vi "Live Capture Functional Stack3.64bit.Test.vi"() -> ()   [LabVIEW 2014]
uses:
  subvis/Stack Track.ctl
  subvis/Stack_State.ctl
  Desktop/camtiff/ctiff.llb/__CTIFFNewFileAndStyleUINT16.vi
  Desktop/camtiff/ctiff.llb/__CTIFFAddNewPageUINT16.vi
panel:
  out "Frame Index":i32
  in  "Temp":path=path "C:/temp.tmp"
  in  "Frames":i32=100
  in  "HardDisk Record":bool
  in  "Internal Line Interval":dbl
  in  "Slit Width / Lines":sgl=150.0
  in  "Camera Readout Mode":u16(ring)=12 items=["Full Frame"=1, "Slit Scanning"=12]
  in  "Readout Direction":sgl(ring)=1.0 items=["Forward"=1, "Backward"=2]
  in  "Trigger Mode":sgl(ring)=1.0 items=["Normal"=1, "Start "=6]
  in  "Trigger Source":sgl(ring)=2.0 items=["Internal"=1, "External"=2]
  out "State":T1=enum."Start Sequence"
  out "Image":u16[][](graph)
  out "Saving":bool
  in  "AutoIncrement":bool=TRUE
  in  "Path":path=path "C:/Users/spim/Desktop/Craig Cap/temp/a.tiff"
  in  "Frames":i32=100
  out "Frame Index":i32
  out "error out":errorcluster
  in  "stop":bool
  in  "Ram Record":bool
  out "Total Frames":i32
  out "Elapsed Time":u32
  out "Software FPS":dbl
  out "Camera FPS":dbl
  in  "H Offset":i32 min=0 max=0 step=4
  in  "H Width":i32 min=0 max=2048 step=4
  out "SMD":dbl
  out "SHO":i32
  in  "V Offset":i32 min=0 max=0 step=4
  in  "V Width":i32 min=0 max=2048 step=4
  in  "Binning":u16(ring) items=["1x1"=1, "2x2"=2, "4x4"=4]
  out "SHW":i32
  out "SVO":i32
  out "SVW":i32
  in  "Scan Mode":dbl min=0.0 max=2.0 step=1.0
  in  "Exposure":dbl min=0.0 max=10.000004210526315 step=1e-08
  out "EXP":dbl
  out "Camera Model":string
  out "Camera Version":string
  out "Camera Serial":string
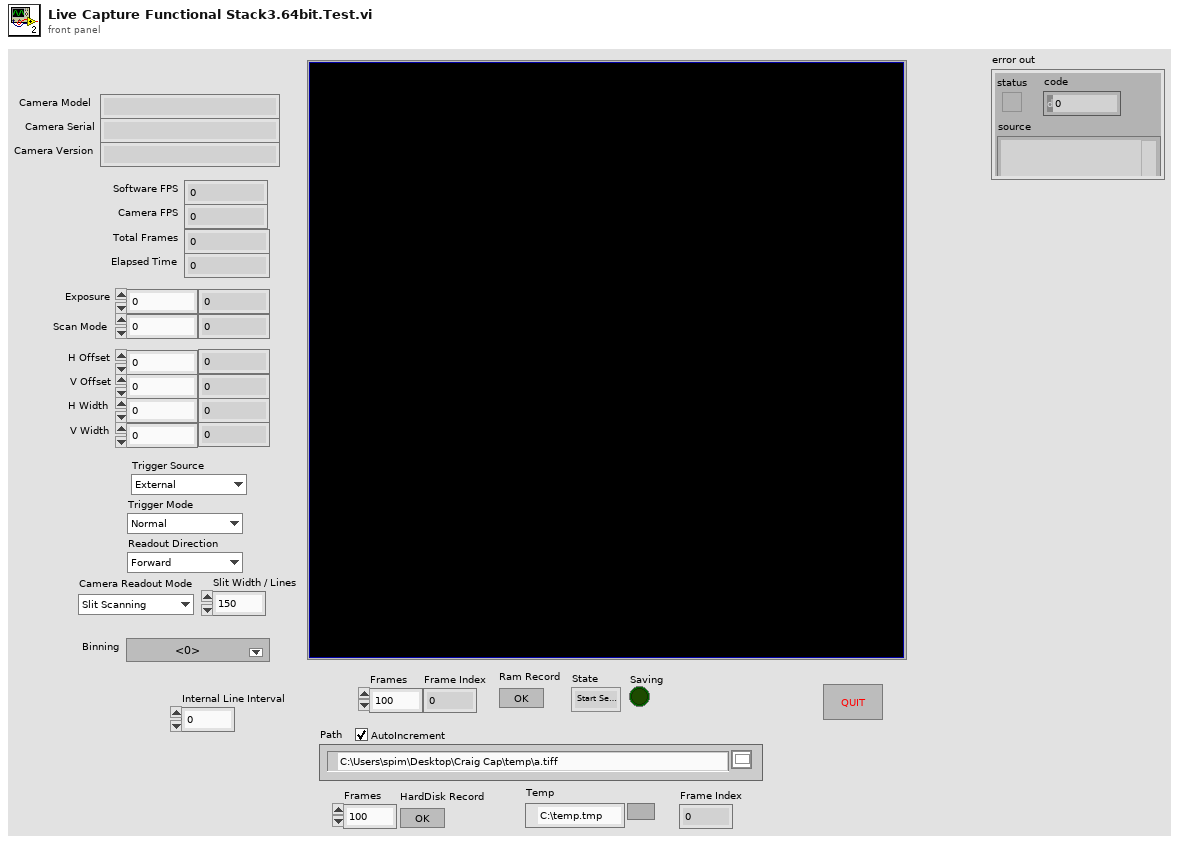
[diagram p1: front panel]
types:
  T1 = typedef "Stack Track.ctl" = enum16{"Idle", "Start Sequence", "Read Disk", "STOP", "Collecting", "End"}
  T2 = enum8{"Enabled", "Disabled", "Disabled and Grayed Out"}
  T3 = typedef "Stack_State.ctl" = cluster{"State":T1, "Stack Number":i32, "Image":u16[][]}
  T4 = cluster{"Model":string, "Camera ID":string, "Firmware":string}
  T5 = cluster{"Value":i32, "Minimum":i32, "Maximum":i32, "Increment":i32}
  T6 = cluster{"height":u32, "width":u32, "datatype":u32}
  T7 = cluster{"H Offset":i32, "V Offset":i32, "H Width":i32, "V Width":i32}
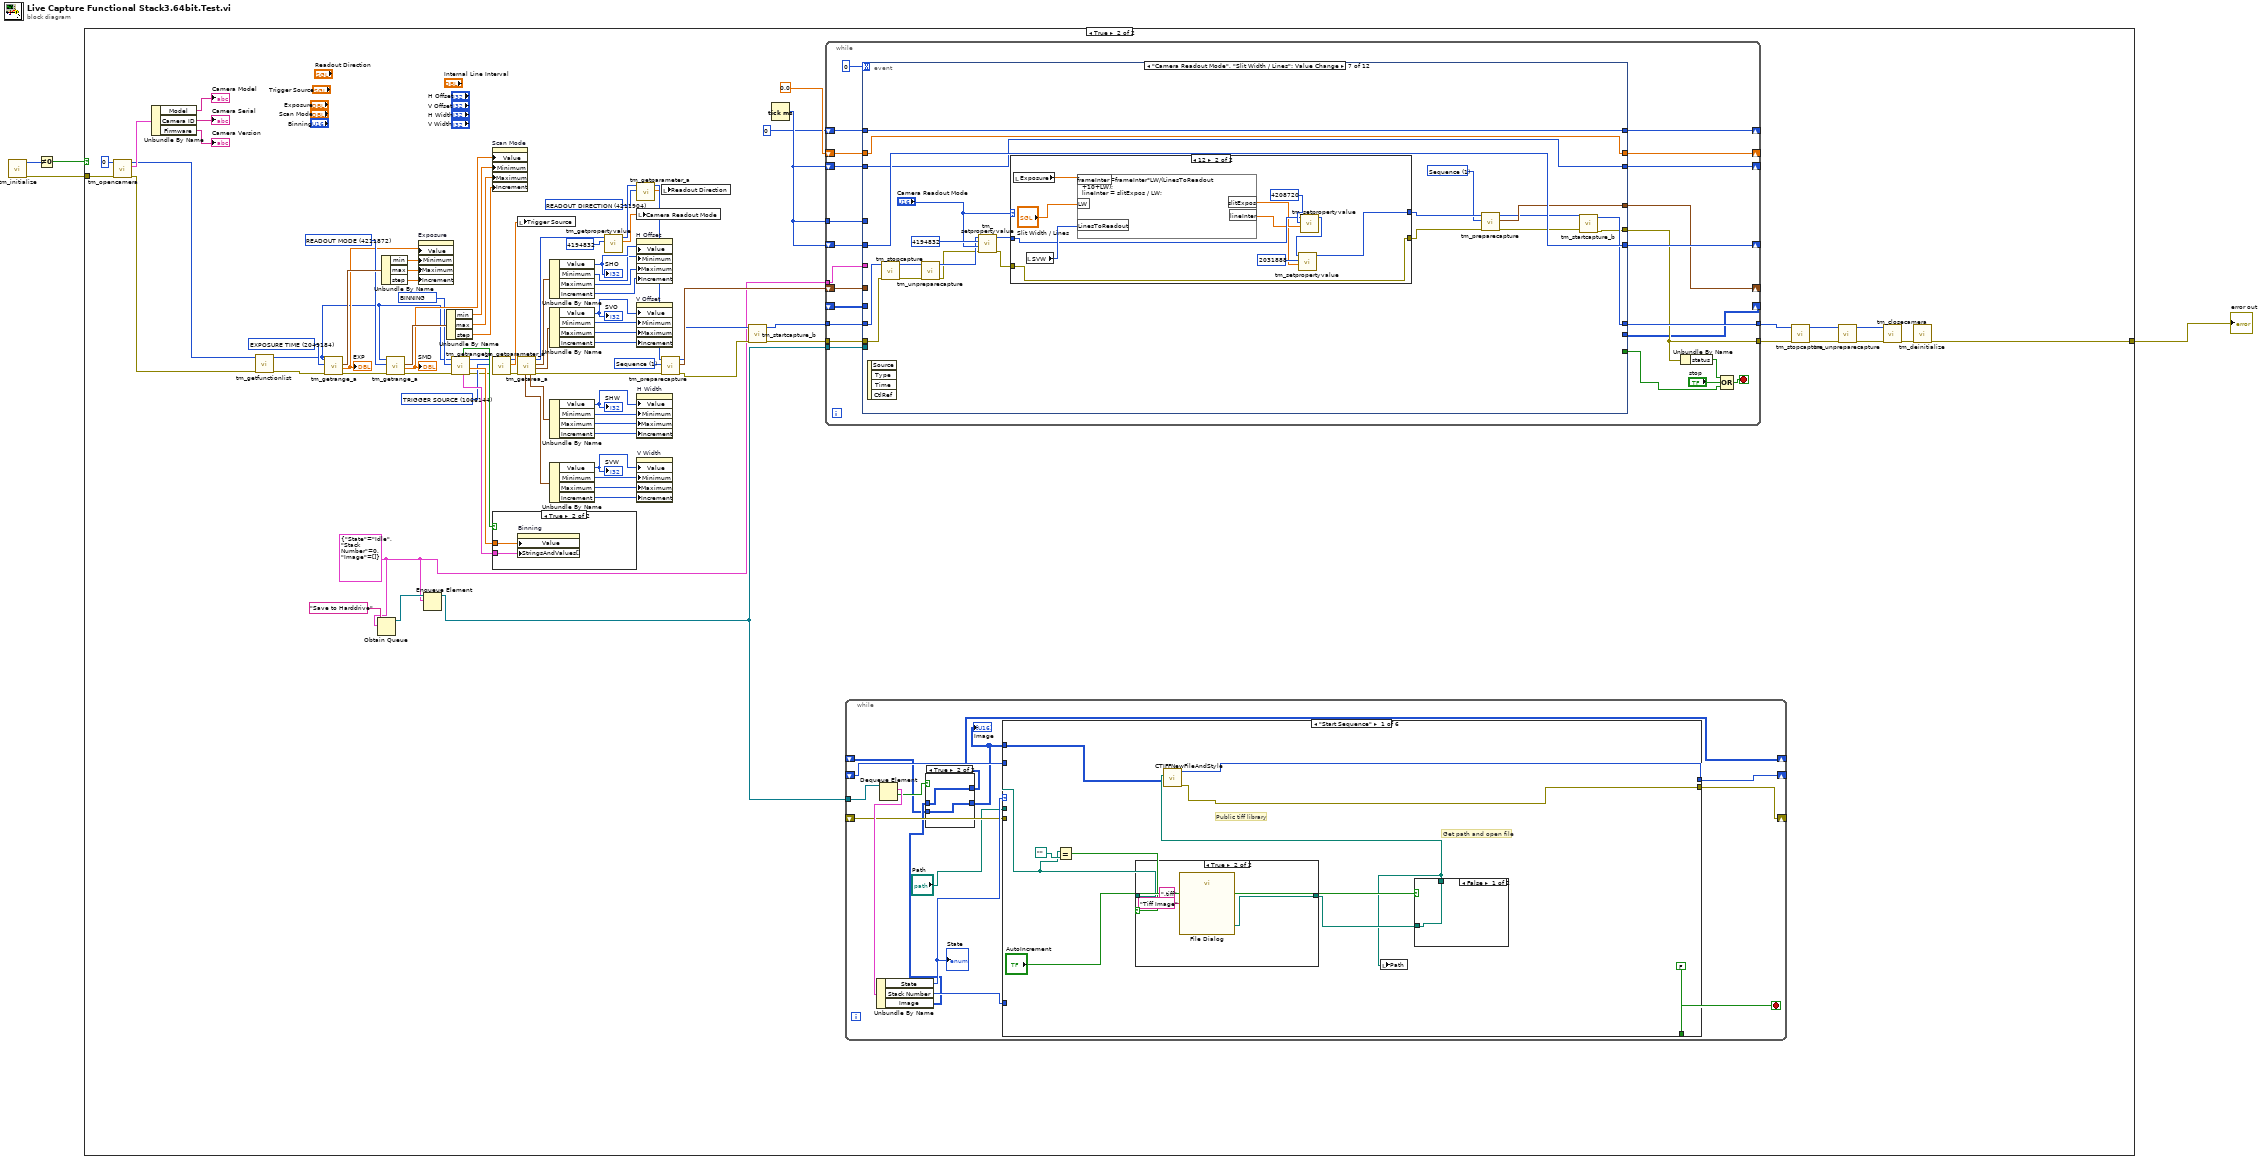
[diagram p0: block diagram]
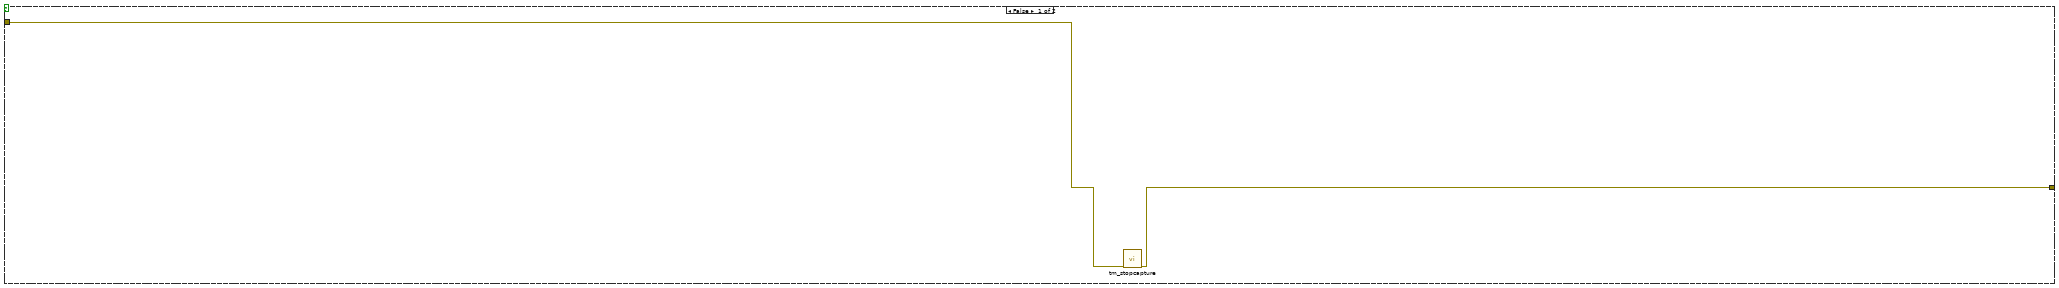
[diagram p2: hidden frame]
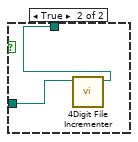
[diagram p5: hidden frame]
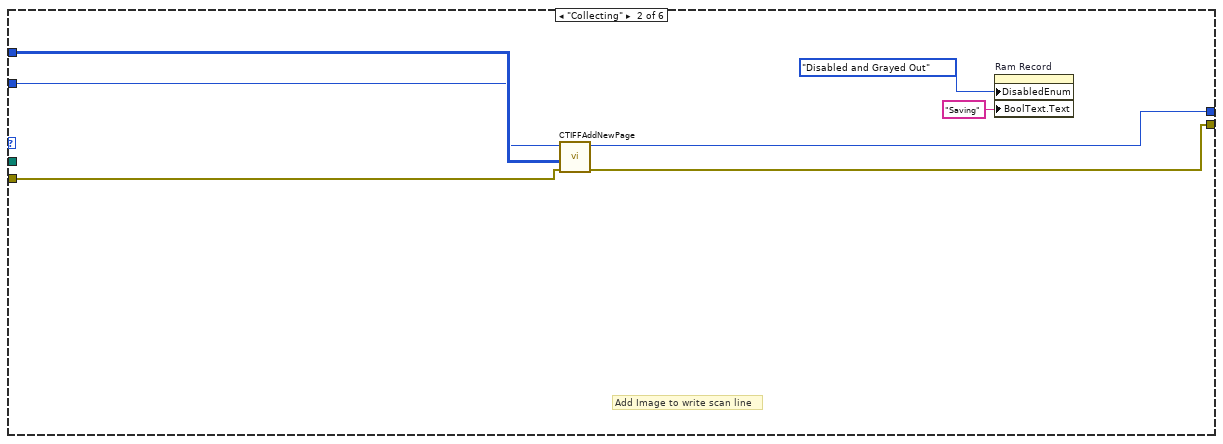
[diagram p6: hidden frame]
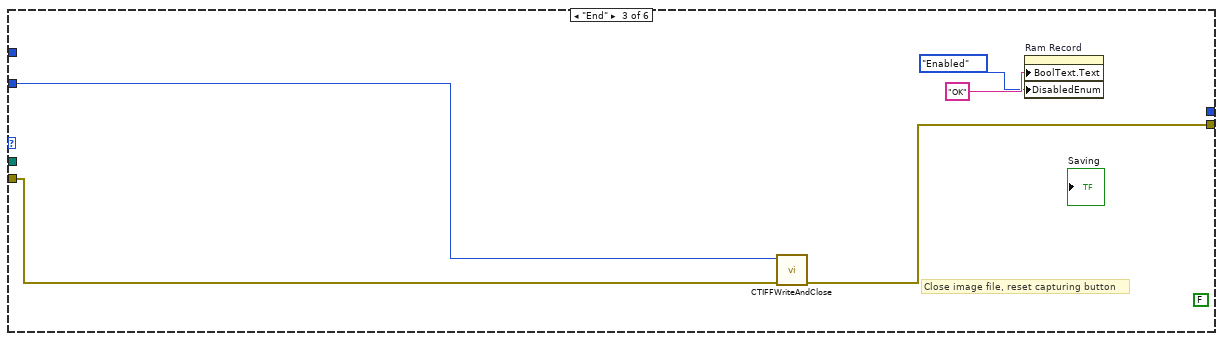
[diagram p7: hidden frame]
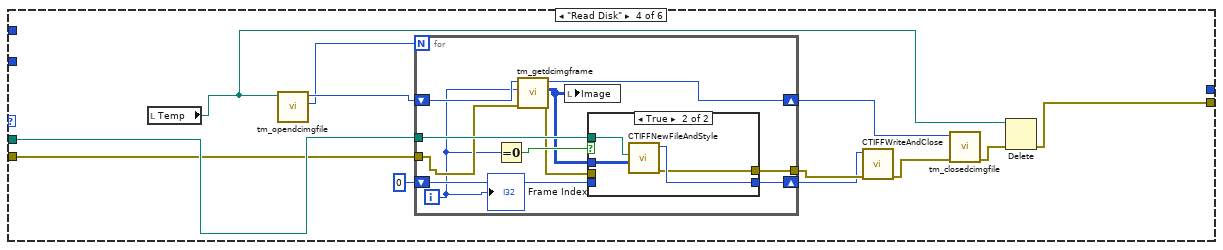
[diagram p8: hidden frame]
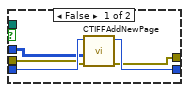
[diagram p9: hidden frame]
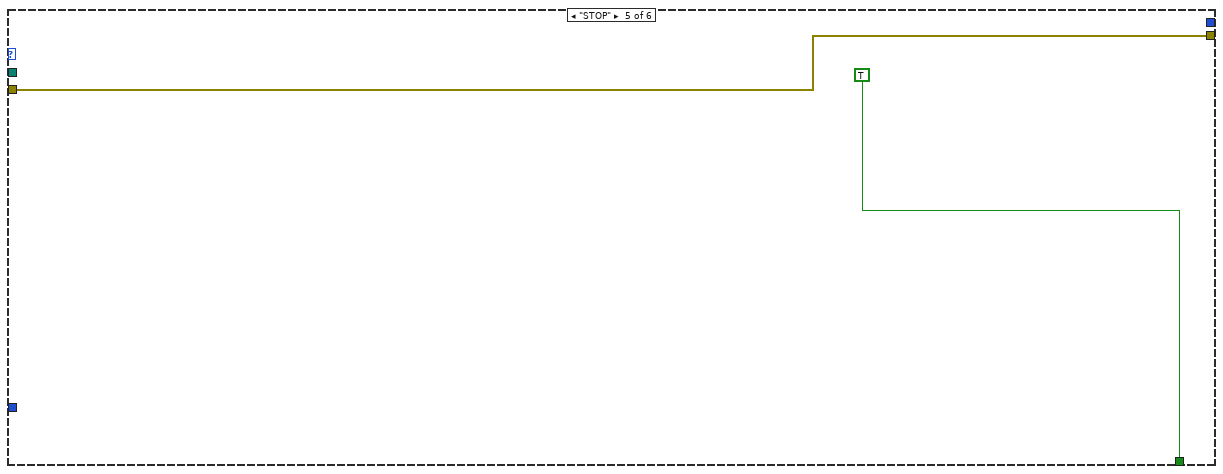
[diagram p10: hidden frame]
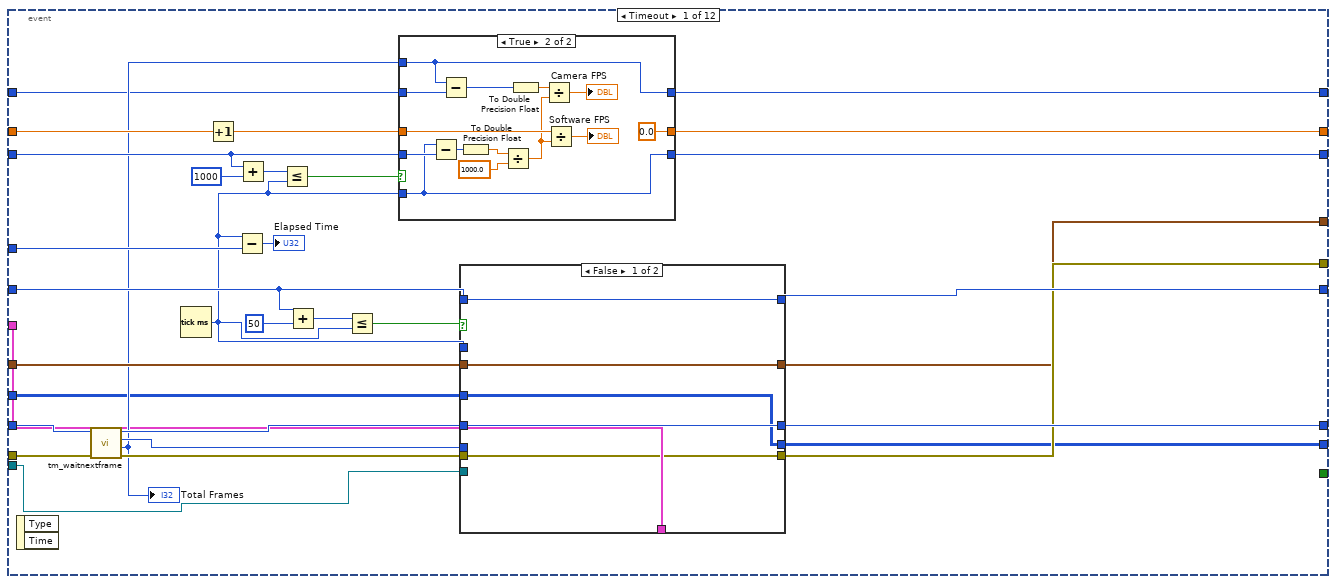
[diagram p13: hidden frame]
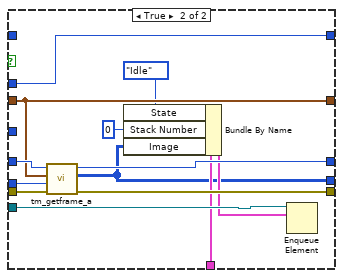
[diagram p15: hidden frame]
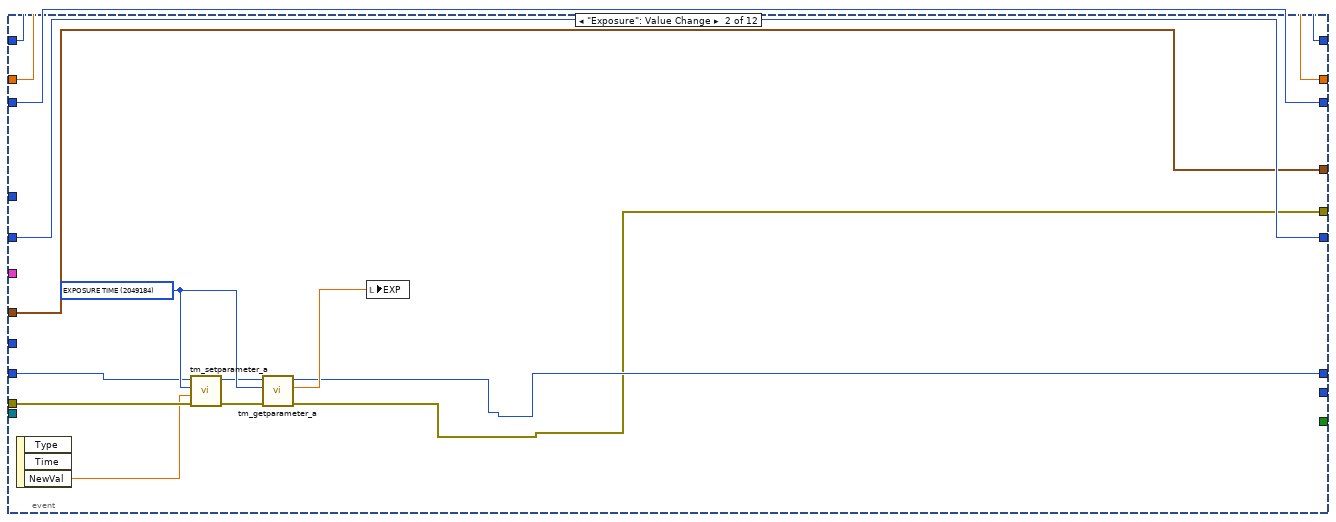
[diagram p16: hidden frame]
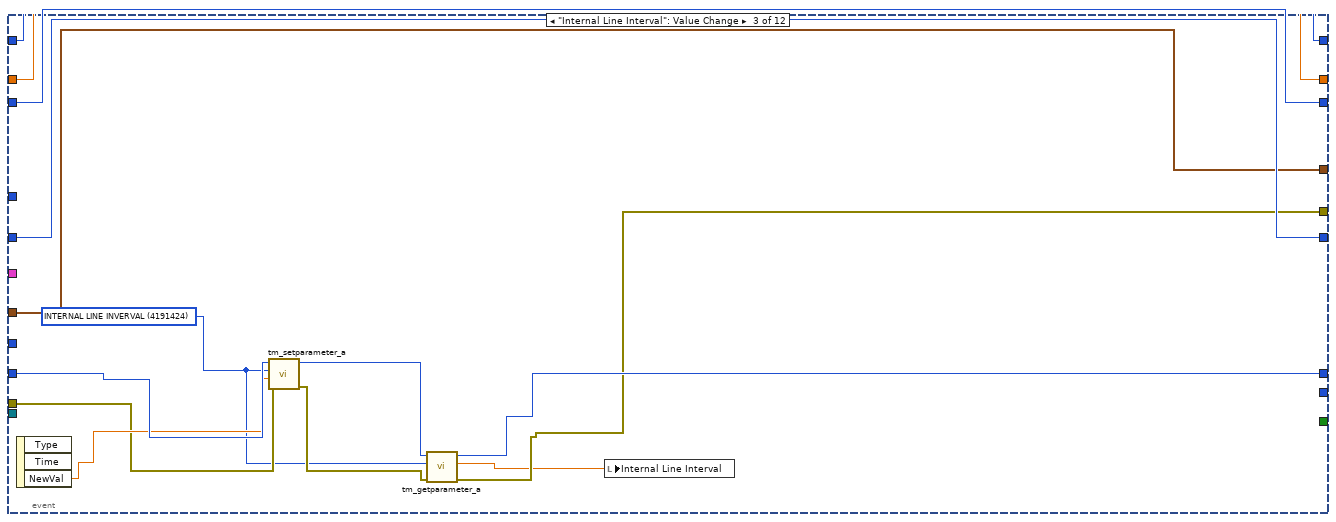
[diagram p17: hidden frame]
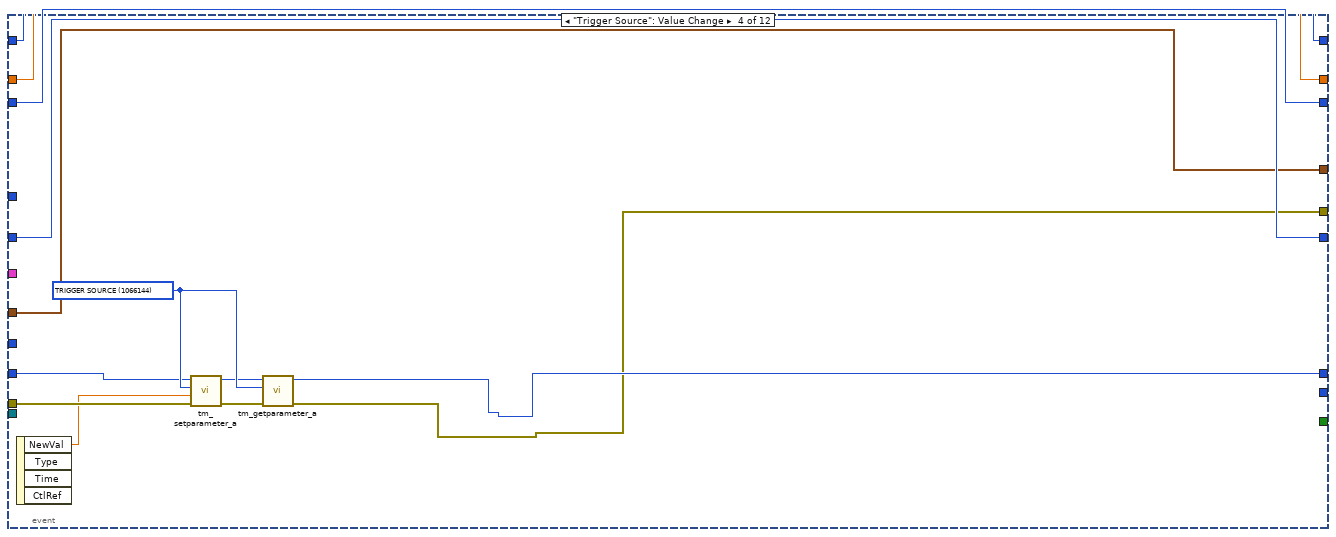
[diagram p18: hidden frame]
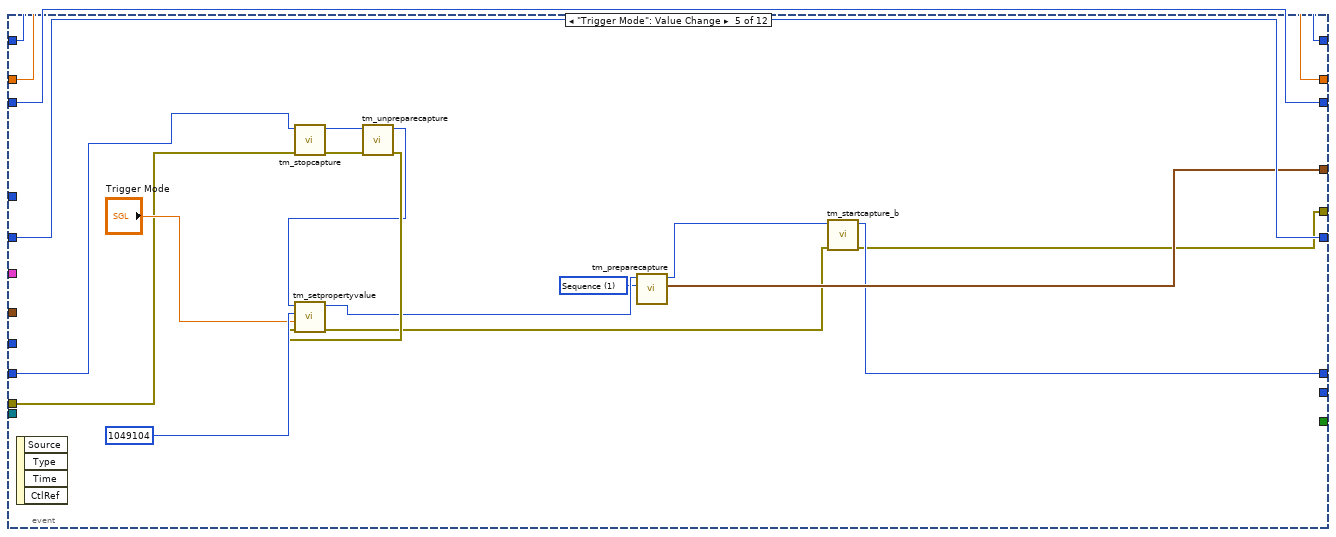
[diagram p19: hidden frame]
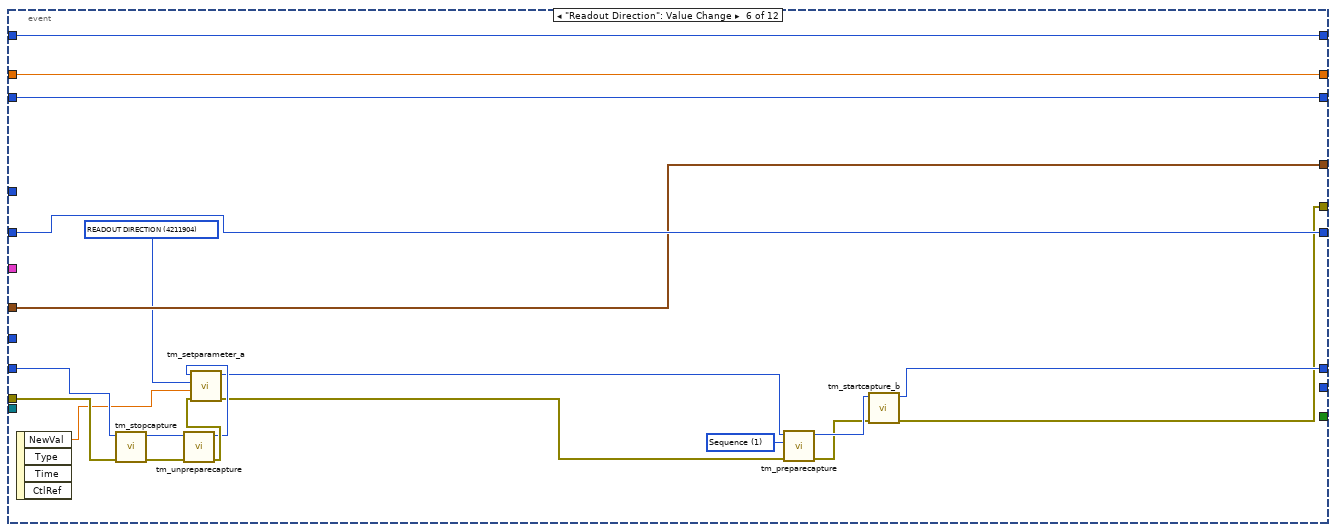
[diagram p20: hidden frame]
diagram:
  n1 = call <userlib>:"tm_initialize.vi"() -> ("error out"=w2:errorcluster, "Number Of Cameras"=w1:u32)  [unwired: 8 in, 2 out]
  n2 = Not Equal To 0?(x=w1) -> (x != 0?=w4:bool)
  n3 = case shown="True" w4 {
    tunnel: [w5 w86] -> w3
    tunnel: w2 -> [w6 w89]
    frame False {
      n4 = call <userlib>:"tm_stopcapture.vi"("error in (no error)"=w6) -> ("error out"=w5:errorcluster)  [unwired: 9 in, 1 out]
    }
    frame True {
      w14 = u32 4211904 items=["SENSOR MODE"=4212128, "CCD MODE"=4212384, "READOUT MODE"=4211872, "ACTIVE VIEW INDEX"=4343136, "BITS PER CHANNEL"=4342976, "IMAGE PIXEL TYPE"=4343296, "BINNING"=4215968, "EXPOSURE TIME"=2049184, "CONTRAST GAIN"=3163312, "CONTRAST OFFSET"=3163328, "LIGHT MODE"=2114720, "SENSITIVITY"=2114992, "PHOTON IMAGING MODE"=2115200, "HIGH DYNAMIC RANGE MODE"=3163360, "WHITE BALANCE"=3163568, "TEMPERATURE"=2115232, "TEMPERATURE TARGET"=2115264, "SENSOR COOLER FAN"=2115296, "LINEBUNDLE HEIGHT"=4212192, "MECHANICAL SHUTTER"=2115488, "BACK FOCUS POSITION"=8422304, "TRIGGER CONNECTOR"=1066432, "TRIGGER SOURCE"=1066144, "OUTPUT TRIGGER SOURCE"=1852576, "TRIGGER GLOBAL EXPOSURE"=2049680, "FIRST TRIGGER BEHAVIOR"=2049696, "CHANNEL SYNC"=1852352, "READOUT DIRECTION"=4211904, "PRE HSYNC COUNT"=1852704] ("Parameter")
      w24 = u32 1066144 items=["SENSOR MODE"=4212128, "CCD MODE"=4212384, "READOUT MODE"=4211872, "ACTIVE VIEW INDEX"=4343136, "BITS PER CHANNEL"=4342976, "IMAGE PIXEL TYPE"=4343296, "BINNING"=4215968, "EXPOSURE TIME"=2049184, "CONTRAST GAIN"=3163312, "CONTRAST OFFSET"=3163328, "LIGHT MODE"=2114720, "SENSITIVITY"=2114992, "PHOTON IMAGING MODE"=2115200, "HIGH DYNAMIC RANGE MODE"=3163360, "WHITE BALANCE"=3163568, "TEMPERATURE"=2115232, "TEMPERATURE TARGET"=2115264, "SENSOR COOLER FAN"=2115296, "LINEBUNDLE HEIGHT"=4212192, "MECHANICAL SHUTTER"=2115488, "BACK FOCUS POSITION"=8422304, "TRIGGER CONNECTOR"=1066432, "TRIGGER SOURCE"=1066144, "OUTPUT TRIGGER SOURCE"=1852576, "TRIGGER GLOBAL EXPOSURE"=2049680, "FIRST TRIGGER BEHAVIOR"=2049696, "CHANNEL SYNC"=1852352, "READOUT DIRECTION"=4211904, "PRE HSYNC COUNT"=1852704] ("Parameter")
      w7 = T3 {"State"=enum."Idle", "Stack Number"=0, "Image"=[]} ("input cluster")
      w32 = u32 2049184 items=["BINNING"=4215968, "BITS PER CHANNEL"=4342976, "ACTIVE VIEW INDEX"=4343136, "CCD MODE"=4212384, "SENSOR MODE"=4212128, "READOUT MODE"=4211872, "EXPOSURE TIME"=2049184, "CONTRAST GAIN"=3163312, "CONTRAST OFFSET"=3163328, "LIGHT MODE"=2114720, "SENSITIVITY"=2114992, "WHITE BALANCE"=3163568, "PHOTON IMAGING MODE"=2115200, "HIGH DYNAMIC RANGE MODE"=3163360, "TRIGGER SOURCE"=1066144, "TRIGGER ACTIVE"=1066160, "TRIGGER MODE"=1066400, "TRIGGER POLARITY"=1066416, "TRIGGER GLOBAL EXPOSURE"=2049680, "FIRST TRIGGER BEHAVIOR"=2049696, "TRIGGER TIMES"=1066448, "OUTPUT TRIGGER POLARITY"=1852592, "OUTPUT TRIGGER DELAY"=1852624, "OUTPUT TRIGGER PERIOD"=1852640, "TEMPERATURE"=2115232, "TEMPERATURE TARGET"=2115264, "SENSOR COOLER FAN"=2115296, "MECHANICAL SHUTTER"=2115488, "BACK FOCUS POSITION"=8422304, "FRAMEBUNDLE MODE"=4346784, "FRAMEBUNDLE NUMBER"=4346800, "LINEBUNDLE HEIGHT"=4212192, "TRIGGER CONNECTOR"=1066432, "IMAGE PIXEL TYPE"=4343296, "OUTPUT TRIGGER KIND"=1852656, "READOUT DIRECTION"=4211904, "CHANNEL SYNC"=1852352] ("Parameter")
      w33 = u32 4211872 items=["BINNING"=4215968, "BITS PER CHANNEL"=4342976, "ACTIVE VIEW INDEX"=4343136, "CCD MODE"=4212384, "SENSOR MODE"=4212128, "READOUT MODE"=4211872, "EXPOSURE TIME"=2049184, "CONTRAST GAIN"=3163312, "CONTRAST OFFSET"=3163328, "LIGHT MODE"=2114720, "SENSITIVITY"=2114992, "WHITE BALANCE"=3163568, "PHOTON IMAGING MODE"=2115200, "HIGH DYNAMIC RANGE MODE"=3163360, "TRIGGER SOURCE"=1066144, "TRIGGER ACTIVE"=1066160, "TRIGGER MODE"=1066400, "TRIGGER POLARITY"=1066416, "TRIGGER GLOBAL EXPOSURE"=2049680, "FIRST TRIGGER BEHAVIOR"=2049696, "TRIGGER TIMES"=1066448, "OUTPUT TRIGGER POLARITY"=1852592, "OUTPUT TRIGGER DELAY"=1852624, "OUTPUT TRIGGER PERIOD"=1852640, "TEMPERATURE"=2115232, "TEMPERATURE TARGET"=2115264, "SENSOR COOLER FAN"=2115296, "MECHANICAL SHUTTER"=2115488, "BACK FOCUS POSITION"=8422304, "FRAMEBUNDLE MODE"=4346784, "FRAMEBUNDLE NUMBER"=4346800, "LINEBUNDLE HEIGHT"=4212192, "TRIGGER CONNECTOR"=1066432, "IMAGE PIXEL TYPE"=4343296, "OUTPUT TRIGGER KIND"=1852656, "READOUT DIRECTION"=4211904, "CHANNEL SYNC"=1852352] ("Parameter")
      w34 = u32 4215968 items=["BINNING"=4215968, "BITS PER CHANNEL"=4342976, "ACTIVE VIEW INDEX"=4343136, "CCD MODE"=4212384, "SENSOR MODE"=4212128, "READOUT MODE"=4211872, "EXPOSURE TIME"=2049184, "CONTRAST GAIN"=3163312, "CONTRAST OFFSET"=3163328, "LIGHT MODE"=2114720, "SENSITIVITY"=2114992, "WHITE BALANCE"=3163568, "PHOTON IMAGING MODE"=2115200, "HIGH DYNAMIC RANGE MODE"=3163360, "TRIGGER SOURCE"=1066144, "TRIGGER ACTIVE"=1066160, "TRIGGER MODE"=1066400, "TRIGGER POLARITY"=1066416, "TRIGGER GLOBAL EXPOSURE"=2049680, "FIRST TRIGGER BEHAVIOR"=2049696, "TRIGGER TIMES"=1066448, "OUTPUT TRIGGER POLARITY"=1852592, "OUTPUT TRIGGER DELAY"=1852624, "OUTPUT TRIGGER PERIOD"=1852640, "TEMPERATURE"=2115232, "TEMPERATURE TARGET"=2115264, "SENSOR COOLER FAN"=2115296, "MECHANICAL SHUTTER"=2115488, "BACK FOCUS POSITION"=8422304, "FRAMEBUNDLE MODE"=4346784, "FRAMEBUNDLE NUMBER"=4346800, "LINEBUNDLE HEIGHT"=4212192, "TRIGGER CONNECTOR"=1066432, "IMAGE PIXEL TYPE"=4343296, "OUTPUT TRIGGER KIND"=1852656, "READOUT DIRECTION"=4211904, "CHANNEL SYNC"=1852352] ("Parameter")
      w84 = 1 items=["Snap", "Sequence"] ("Capture mode")
      n5 = call <userlib>:"tm_opencamera.vi"("error in (no error)"=w89, "Camera Index"=u32 0) -> ("error out"=w28:errorcluster, "Camera Details"=w46:T4, "Handle out"=w12:u32)  [unwired: 7 in]
      n6 = Unbundle By Name(w46) -> ("Model"=→"Camera Model":string, "Camera ID"=→"Camera Serial":string, "Firmware"=→"Camera Version":string)
      n7 = call <userlib>:"tm_getfunctionlist.vi"("error in (no error)"=w28, "Handle in"=w12) -> ("error out"=w27:errorcluster, "Handle out"=w29:u32)  [unwired: 7 in, 1 out]
      n8 = call <userlib>:"tm_getrange_a.vi"("error in (no error)"=w27, "Parameter"=w32, "Handle in"=w29) -> ("error out"=w41:errorcluster, "default"=w30:dbl, "Range"=w42:cluster{"min":dbl, "max":dbl, "step":dbl})  [unwired: 2 in, 4 out]
      "EXP" <- w30
      n9 = Obtain Queue(name (unnamed)="Save to Harddrive", element data type=w7) -> (queue out=w9:refnum<queue>)  [unwired: 3 in, 2 out]
      n10 = Unbundle By Name(w42) -> ("min"=w79:dbl, "max"=w78:dbl, "step"=w77:dbl)
      n11 = call <userlib>:"tm_getrange_a.vi"("error in (no error)"=w41, "Parameter"=w33, "Handle in"=w29) -> ("error out"=w38:errorcluster, "default"=w39:dbl, "Range"=w40:cluster{"min":dbl, "max":dbl, "step":dbl})  [unwired: 2 in, 4 out]
      "SMD" <- w39
      n12 = property on="Exposure" class="DigNum (strict)"("Value"=w30, "Minimum"=w79, "Maximum"=w78, "Increment"=w77) -> ()  [unwired: 2 in, 2 out]
      n13 = Enqueue Element(queue=w9, element=w7) -> (queue out=w8:refnum<queue>)  [unwired: 2 in, 2 out]
      n14 = Unbundle By Name(w40) -> ("min"=w76:dbl, "max"=w75:dbl, "step"=w74:dbl)
      n15 = call <userlib>:"tm_getrange_a.vi"("error in (no error)"=w38, "Parameter"=w34, "Handle in"=w29) -> ("error out"=w21:errorcluster, "default"=w36:dbl, "Handle out"=w23:u32, "Value Names"=w35:cluster{"Name":string, "Value":dbl}[], "Writable"=w37:bool)  [unwired: 2 in, 2 out]
      n16 = property on="Scan Mode" class="DigNum (strict)"("Value"=w39, "Minimum"=w76, "Maximum"=w75, "Increment"=w74) -> ()  [unwired: 2 in, 2 out]
      n17 = call <userlib>:"tm_getparameter_a.vi"("error in (no error)"=w21, "Parameter"=w24, "Handle in"=w23) -> ("error out"=w20:errorcluster, "Value out"=w25:dbl, "Handle out"=w22:u32)  [unwired: 6 in]
      n18 = case shown="True" w37 {
        tunnel: w35 -> [_ w174]
        tunnel: w36 -> [_ w173]
        frame False {
        }
        frame True {
          n19 = property on="Binning" class="Ring (strict)"("Value"=w173, "StringsAndValues[]"=w174) -> ()  [unwired: 2 in, 2 out]
        }
      }
      n20 = local write "Trigger Source"(w25) -> ()
      n21 = call <userlib>:"tm_getarea_a.vi"("error in (no error)"=w20, "Handle in"=w22) -> ("error out"=w26:errorcluster, "V Offset"=w73:T5, "H Offset"=w52:T5, "Handle out"=w17:u32, "H Width"=w72:T5, "V Width"=w71:T5)  [unwired: 4 in]
      n22 = Unbundle By Name(w52) -> ("Value"=w51:i32, "Minimum"=w50:i32, "Maximum"=w49:i32, "Increment"=w48:i32)
      "SHO" <- w51
      n23 = Unbundle By Name(w73) -> ("Value"=w61:i32, "Minimum"=w70:i32, "Maximum"=w69:i32, "Increment"=w68:i32)
      "SVO" <- w61
      n24 = Unbundle By Name(w72) -> ("Value"=w60:i32, "Minimum"=w67:i32, "Maximum"=w66:i32, "Increment"=w65:i32)
      "SHW" <- w60
      n25 = Unbundle By Name(w71) -> ("Value"=w59:i32, "Minimum"=w64:i32, "Maximum"=w63:i32, "Increment"=w62:i32)
      "SVW" <- w59
      n26 = call <userlib>:"tm_getpropertyvalue.vi"("Property ID"=u32 4194832, "Handle in"=w17) -> ("Value in"=w18:sgl, "Handle out"=w16:u32)  [unwired: 7 in, 1 out]
      n27 = call <userlib>:"tm_getparameter_a.vi"("Parameter"=w14, "Handle in"=w16) -> ("Value out"=w13:dbl, "Handle out"=w15:u32)  [unwired: 7 in, 1 out]
      n28 = local write "Camera Readout Mode"(w18) -> ()
      n29 = property on="H Offset" class="DigNum (strict)"("Value"=w51, "Minimum"=w50, "Maximum"=w49, "Increment"=w48) -> ()  [unwired: 2 in, 2 out]
      n30 = property on="V Offset" class="DigNum (strict)"("Value"=w61, "Minimum"=w70, "Maximum"=w69, "Increment"=w68) -> ()  [unwired: 2 in, 2 out]
      n31 = property on="H Width" class="DigNum (strict)"("Value"=w60, "Minimum"=w67, "Maximum"=w66, "Increment"=w65) -> ()  [unwired: 2 in, 2 out]
      n32 = property on="V Width" class="DigNum (strict)"("Value"=w59, "Minimum"=w64, "Maximum"=w63, "Increment"=w62) -> ()  [unwired: 2 in, 2 out]
      n33 = local write "Readout Direction"(w13) -> ()
      n34 = call <userlib>:"tm_preparecapture.vi"("error in (no error)"=w26, "Capture mode"=w84, "Handle in"=w15) -> ("error out"=w10:errorcluster, "Buffer Info"=w81:T6, "Handle out"=w11:u32)  [unwired: 5 in, 1 out]
      n35 = call <userlib>:"tm_startcapture_b.vi"("error in (no error)"=w10, "Handle in"=w11) -> ("error out"=w83:errorcluster, "Handle out"=w82:u32)  [unwired: 8 in]
      n36 = Tick Count (ms)() -> (millisecond timer value=w80:u32)
      n37 = while {
        tunnel: w83 -> [w187]
        tunnel: [w185] -> w58
        tunnel: [w184] -> w57
        shift-right: [w194] -> _
        shift-left: w80 -> [w192]
        shift-right: [w195] -> _
        shift-left: 0.0 -> [w193]
        shift-right: [w186] -> _
        shift-left: w80 -> [w190]
        tunnel: w82 -> [w188]
        tunnel: w80 -> [w191]
        shift-right: [w183] -> _
        shift-left: w81 -> [w189]
        shift-right: [w180] -> _
        shift-left: 0 -> [w181]
        tunnel: w8 -> [w179]
        shift-right: [w177] -> _
        shift-left: _ -> [w176]
        tunnel: w7 -> [w175]
        stop <- w196 stop-if-true
        n38 = event shown="[6] \"Camera Readout Mode\", \"Slit Width / Lines\": Value Change" {
          selector: _ -> [_ _ _ _ _ _ _ _ _ _ _ _]
          dyn-events: _ -> [_ _ _ _ _ _ _ _ _ _ _ _]
          timeout: 0 -> [_ _ _ _ _ _ _ _ _ _ _ _]
          tunnel: [w208 w277 w291 w304 w323 w343 w365 w393 w490 w584 w620 w665] -> w195
          tunnel: [w207 w278 w292 w305 w324 w344 w366 w394 w491 w585 w621 w666] -> w194
          tunnel: w193 -> [w219 w277 w291 w304 w323 w343 w365 w393 w490 w584 w620 w665]
          tunnel: w192 -> [w210 w278 w292 w305 w324 w344 w366 w394 w491 w585 w621 w666]
          tunnel: w191 -> [w215 _ _ _ _ _ _ _ _ _ _ _]
          tunnel: w190 -> [w220 w279 w293 w306 w325 w345 w367 w389 w486 w586 w628 w673]
          tunnel: w189 -> [w214 w276 w290 w303 _ w342 _ w390 w487 _ _ _]
          tunnel: w188 -> [w222 w271 w285 w299 w317 w336 w358 w397 w494 w581 w597 w635]
          tunnel: w187 -> [w221 w273 w281 w300 w316 w339 w357 w398 w495 w580 w596 w634]
          tunnel: [w218 w279 w293 w306 w325 w345 w367 w389 w486 w586 w628 w673] -> w186
          tunnel: [w217 w267 w288 w296 w308 w329 w348 w395 w492 w575 w623 w668] -> w185
          tunnel: [w216 w266 w287 w295 w307 w328 w346 w396 w493 w576 w624 w669] -> w184
          tunnel: [w213 w276 w290 w303 w311 w342 w353 w391 w488 w574 w622 w667] -> w183
          tunnel: w181 -> [w205 w275 w289 w302 w322 w341 w364 w392 w489 w573 w593 w629]
          tunnel: [w204 w275 w289 w302 w322 w341 w364 w392 w489 w573 w593 w629] -> w180
          tunnel: w179 -> [w199 _ _ _ _ _ _ w388 w485 _ _ _]
          tunnel: [_ _ _ _ _ _ _ w387 w484 _ _ _] -> w178
          tunnel: w175 -> [w202 _ _ _ _ _ _ w385 _ _ _ _]
          tunnel: [w201 _ _ _ _ _ _ _ _ _ _ _] -> w177
          tunnel: w176 -> [w200 _ _ _ _ _ _ w386 _ _ _ _]
          event Timeout {
            n39 = event-data() -> ()  [unwired: 1 in, 2 out]
            n40 = call <userlib>:"tm_waitnextframe.vi"("error in (no error)"=w221, "Handle in"=w222) -> ("error out"=w225:errorcluster, "Frame Count"=w206:i32, "Frame Index"=w224:i32, "Handle out"=w226:u32)  [unwired: 6 in]
            "Total Frames" <- w206
            n41 = Tick Count (ms)() -> (millisecond timer value=w212:u32)
            n42 = Increment(x=w219) -> (x+1=w209:dbl)
            n43 = Subtract(x=w212, y=w215) -> (x-y=→"Elapsed Time":u32)
            n44 = Add(x=w210, y=u32 1000) -> (x+y=w230:u32)
            n45 = Less Or Equal?(x=w230, y=w212) -> (x <= y?=w211:bool)
            n46 = Add(x=w220, y=u32 50) -> (x+y=w228:u32)
            n47 = Less Or Equal?(x=w228, y=w212) -> (x <= y?=w203:bool)
            n48 = case shown="True" w211 {
              tunnel: w210 -> [w233 w242]
              tunnel: [w233 w239] -> w207
              tunnel: w209 -> [w232 w245]
              tunnel: w212 -> [_ w239]
              tunnel: [w232 0.0] -> w208
              tunnel: w206 -> [_ w234]
              tunnel: w205 -> [w231 w237]
              tunnel: [w231 w234] -> w204
              frame False {
              }
              frame True {
                n49 = Subtract(x=w239, y=w242) -> (x-y=w241:u32)
                n50 = Subtract(x=w234, y=w237) -> (x-y=w235:i32)
                n51 = To Double Precision Float(number=w241) -> (double precision float=w247:dbl)
                n52 = Divide(x=w247, y=1000.0) -> (x/y=w238:dbl)
                n53 = To Double Precision Float(number=w235) -> (double precision float=w236:dbl)
                n54 = Divide(x=w236, y=w238) -> (x/y=→"Camera FPS":dbl)
                n55 = Divide(x=w245, y=w238) -> (x/y=→"Software FPS":dbl)
              }
            }
            n56 = case shown="False" w203 {
              tunnel: w220 -> [w252 _]
              tunnel: w212 -> [_ w265]
              tunnel: [w252 w265] -> w218
              tunnel: w226 -> [w251 w264]
              tunnel: w214 -> [w249 w259]
              tunnel: w225 -> [w250 w263]
              tunnel: [w251 w262] -> w217
              tunnel: [w250 w261] -> w216
              tunnel: w224 -> [_ w260]
              tunnel: [w249 w259] -> w213
              tunnel: w199 -> [_ w258]
              tunnel: w202 -> [_ w254]
              tunnel: [w248 w253] -> w201
              tunnel: w200 -> [w248 _]
              frame False {
              }
              frame True {
                n57 = call <userlib>:"tm_getframe_a.vi"("error in (no error)"=w263, "Frame Index"=w260, "Buffer Info"=w259, "Handle in"=w264) -> ("error out"=w261:errorcluster, "Data 16"=w253:u16[][], "Handle out"=w262:u32)  [unwired: 3 in, 2 out]
                n58 = Bundle By Name(cluster=w254, "State"=Stack_Track."Idle", "Stack Number"=0, "Image"=w253) -> (w255:T3)
                n59 = Enqueue Element(queue=w258, element=w255) -> ()  [unwired: 2 in, 3 out]
              }
            }
          }
          event "Exposure": Value Change {
            w274 = u32 2049184 items=["SENSOR MODE"=4212128, "CCD MODE"=4212384, "READOUT MODE"=4211872, "ACTIVE VIEW INDEX"=4343136, "BITS PER CHANNEL"=4342976, "IMAGE PIXEL TYPE"=4343296, "BINNING"=4215968, "EXPOSURE TIME"=2049184, "CONTRAST GAIN"=3163312, "CONTRAST OFFSET"=3163328, "LIGHT MODE"=2114720, "SENSITIVITY"=2114992, "PHOTON IMAGING MODE"=2115200, "HIGH DYNAMIC RANGE MODE"=3163360, "WHITE BALANCE"=3163568, "TEMPERATURE"=2115232, "TEMPERATURE TARGET"=2115264, "SENSOR COOLER FAN"=2115296, "LINEBUNDLE HEIGHT"=4212192, "MECHANICAL SHUTTER"=2115488, "BACK FOCUS POSITION"=8422304, "TRIGGER CONNECTOR"=1066432, "TRIGGER SOURCE"=1066144, "OUTPUT TRIGGER SOURCE"=1852576, "TRIGGER GLOBAL EXPOSURE"=2049680, "FIRST TRIGGER BEHAVIOR"=2049696, "CHANNEL SYNC"=1852352, "READOUT DIRECTION"=4211904, "PRE HSYNC COUNT"=1852704] ("Parameter")
            n60 = event-data() -> ("NewVal"=w272:dbl)  [unwired: 1 in, 2 out]
            n61 = call <userlib>:"tm_setparameter_a.vi"("error in (no error)"=w273, "Value in"=w272, "Parameter"=w274, "Handle in"=w271) -> ("error out"=w270:errorcluster, "Handle out"=w269:u32)  [unwired: 6 in]
            n62 = call <userlib>:"tm_getparameter_a.vi"("error in (no error)"=w270, "Parameter"=w274, "Handle in"=w269) -> ("error out"=w266:errorcluster, "Value out"=w268:dbl, "Handle out"=w267:u32)  [unwired: 6 in]
            n63 = local write "EXP"(w268) -> ()
          }
          event "Internal Line Interval": Value Change {
            w280 = u32 4191424 items=["SENSOR MODE"=4212128, "CCD MODE"=4212384, "READOUT MODE"=4211872, "ACTIVE VIEW INDEX"=4343136, "BITS PER CHANNEL"=4342976, "IMAGE PIXEL TYPE"=4343296, "BINNING"=4215968, "EXPOSURE TIME"=2049184, "CONTRAST GAIN"=3163312, "CONTRAST OFFSET"=3163328, "LIGHT MODE"=2114720, "SENSITIVITY"=2114992, "PHOTON IMAGING MODE"=2115200, "HIGH DYNAMIC RANGE MODE"=3163360, "WHITE BALANCE"=3163568, "TEMPERATURE"=2115232, "TEMPERATURE TARGET"=2115264, "SENSOR COOLER FAN"=2115296, "LINEBUNDLE HEIGHT"=4212192, "MECHANICAL SHUTTER"=2115488, "BACK FOCUS POSITION"=8422304, "TRIGGER CONNECTOR"=1066432, "TRIGGER SOURCE"=1066144, "OUTPUT TRIGGER SOURCE"=1852576, "TRIGGER GLOBAL EXPOSURE"=2049680, "FIRST TRIGGER BEHAVIOR"=2049696, "CHANNEL SYNC"=1852352, "READOUT DIRECTION"=4211904, "PRE HSYNC COUNT"=1852704, "INTERNAL LINE SPEED"=4191408, "INTERNAL LINE INVERVAL"=4191424] ("Parameter")
            n64 = event-data() -> ("NewVal"=w284:dbl)  [unwired: 1 in, 2 out]
            n65 = call <userlib>:"tm_setparameter_a.vi"("error in (no error)"=w281, "Value in"=w284, "Parameter"=w280, "Handle in"=w285) -> ("error out"=w282:errorcluster, "Handle out"=w283:u32)  [unwired: 6 in]
            n66 = call <userlib>:"tm_getparameter_a.vi"("error in (no error)"=w282, "Parameter"=w280, "Handle in"=w283) -> ("error out"=w287:errorcluster, "Value out"=w286:dbl, "Handle out"=w288:u32)  [unwired: 6 in]
            n67 = local write "Internal Line Interval"(w286) -> ()
          }
          event "Trigger Source": Value Change {
            w301 = u32 1066144 items=["SENSOR MODE"=4212128, "CCD MODE"=4212384, "READOUT MODE"=4211872, "ACTIVE VIEW INDEX"=4343136, "BITS PER CHANNEL"=4342976, "IMAGE PIXEL TYPE"=4343296, "BINNING"=4215968, "EXPOSURE TIME"=2049184, "CONTRAST GAIN"=3163312, "CONTRAST OFFSET"=3163328, "LIGHT MODE"=2114720, "SENSITIVITY"=2114992, "PHOTON IMAGING MODE"=2115200, "HIGH DYNAMIC RANGE MODE"=3163360, "WHITE BALANCE"=3163568, "TEMPERATURE"=2115232, "TEMPERATURE TARGET"=2115264, "SENSOR COOLER FAN"=2115296, "LINEBUNDLE HEIGHT"=4212192, "MECHANICAL SHUTTER"=2115488, "BACK FOCUS POSITION"=8422304, "TRIGGER CONNECTOR"=1066432, "TRIGGER SOURCE"=1066144, "OUTPUT TRIGGER SOURCE"=1852576, "TRIGGER GLOBAL EXPOSURE"=2049680, "FIRST TRIGGER BEHAVIOR"=2049696, "CHANNEL SYNC"=1852352, "READOUT DIRECTION"=4211904, "PRE HSYNC COUNT"=1852704] ("Parameter")
            n68 = event-data() -> ("NewVal"=w294:sgl)  [unwired: 1 in, 3 out]
            n69 = call <userlib>:"tm_setparameter_a.vi"("error in (no error)"=w300, "Value in"=w294, "Parameter"=w301, "Handle in"=w299) -> ("error out"=w298:errorcluster, "Handle out"=w297:u32)  [unwired: 6 in]
            n70 = call <userlib>:"tm_getparameter_a.vi"("error in (no error)"=w298, "Parameter"=w301, "Handle in"=w297) -> ("error out"=w295:errorcluster, "Handle out"=w296:u32)  [unwired: 6 in, 1 out]
          }
          event "Trigger Mode": Value Change {
            w312 = 1 items=["Snap", "Sequence"] ("Capture mode")
            n71 = event-data() -> ()  [unwired: 1 in, 4 out]
            n72 = call <userlib>:"tm_stopcapture.vi"("error in (no error)"=w316, "Handle in"=w317) -> ("error out"=w319:errorcluster, "Handle out"=w318:u32)  [unwired: 8 in]
            n73 = call <userlib>:"tm_unpreparecapture.vi"("error in (no error)"=w319, "Handle in"=w318) -> ("error out"=w315:errorcluster, "Handle out"=w314:u32)  [unwired: 8 in]
            n74 = call <userlib>:"tm_setpropertyvalue.vi"("error in (no error)"=w315, "Value in"="Trigger Mode", "Property ID"=u32 1049104, "Handle in"=w314) -> ("error out"=w310:errorcluster, "Handle out"=w313:u32)  [unwired: 6 in]
            n75 = call <userlib>:"tm_preparecapture.vi"("Capture mode"=w312, "Handle in"=w313) -> ("Buffer Info"=w311:T6, "Handle out"=w309:u32)  [unwired: 6 in, 2 out]
            n76 = call <userlib>:"tm_startcapture_b.vi"("error in (no error)"=w310, "Handle in"=w309) -> ("error out"=w307:errorcluster, "Handle out"=w308:u32)  [unwired: 8 in]
          }
          event "Readout Direction": Value Change {
            w334 = 1 items=["Snap", "Sequence"] ("Capture mode")
            w327 = u32 4211904 items=["SENSOR MODE"=4212128, "CCD MODE"=4212384, "READOUT MODE"=4211872, "ACTIVE VIEW INDEX"=4343136, "BITS PER CHANNEL"=4342976, "IMAGE PIXEL TYPE"=4343296, "BINNING"=4215968, "EXPOSURE TIME"=2049184, "CONTRAST GAIN"=3163312, "CONTRAST OFFSET"=3163328, "LIGHT MODE"=2114720, "SENSITIVITY"=2114992, "PHOTON IMAGING MODE"=2115200, "HIGH DYNAMIC RANGE MODE"=3163360, "WHITE BALANCE"=3163568, "TEMPERATURE"=2115232, "TEMPERATURE TARGET"=2115264, "SENSOR COOLER FAN"=2115296, "LINEBUNDLE HEIGHT"=4212192, "MECHANICAL SHUTTER"=2115488, "BACK FOCUS POSITION"=8422304, "TRIGGER CONNECTOR"=1066432, "TRIGGER SOURCE"=1066144, "OUTPUT TRIGGER SOURCE"=1852576, "TRIGGER GLOBAL EXPOSURE"=2049680, "FIRST TRIGGER BEHAVIOR"=2049696, "CHANNEL SYNC"=1852352, "READOUT DIRECTION"=4211904, "PRE HSYNC COUNT"=1852704] ("Parameter")
            n77 = event-data() -> ("NewVal"=w326:sgl)  [unwired: 1 in, 3 out]
            n78 = call <userlib>:"tm_stopcapture.vi"("error in (no error)"=w339, "Handle in"=w336) -> ("error out"=w340:errorcluster, "Handle out"=w335:u32)  [unwired: 8 in]
            n79 = call <userlib>:"tm_unpreparecapture.vi"("error in (no error)"=w340, "Handle in"=w335) -> ("error out"=w338:errorcluster, "Handle out"=w337:u32)  [unwired: 8 in]
            n80 = call <userlib>:"tm_setparameter_a.vi"("error in (no error)"=w338, "Value in"=w326, "Parameter"=w327, "Handle in"=w337) -> ("error out"=w331:errorcluster, "Handle out"=w330:u32)  [unwired: 6 in]
            n81 = call <userlib>:"tm_preparecapture.vi"("error in (no error)"=w331, "Capture mode"=w334, "Handle in"=w330) -> ("error out"=w332:errorcluster, "Handle out"=w333:u32)  [unwired: 5 in, 2 out]
            n82 = call <userlib>:"tm_startcapture_b.vi"("error in (no error)"=w332, "Handle in"=w333) -> ("error out"=w328:errorcluster, "Handle out"=w329:u32)  [unwired: 8 in]
          }
          event "Camera Readout Mode", "Slit Width / Lines": Value Change {
            w351 = 1 items=["Snap", "Sequence"] ("Capture mode")
            n83 = event-data() -> ()  [unwired: 1 in, 4 out]
            n84 = call <userlib>:"tm_stopcapture.vi"("error in (no error)"=w357, "Handle in"=w358) -> ("error out"=w359:errorcluster, "Handle out"=w355:u32)  [unwired: 8 in]
            n85 = call <userlib>:"tm_unpreparecapture.vi"("error in (no error)"=w359, "Handle in"=w355) -> ("error out"=w350:errorcluster, "Handle out"=w356:u32)  [unwired: 8 in]
            n86 = call <userlib>:"tm_setpropertyvalue.vi"("error in (no error)"=w350, "Value in"="Camera Readout Mode", "Property ID"=u32 4194832, "Handle in"=w356) -> ("error out"=w360:errorcluster, "Handle out"=w361:u32)  [unwired: 6 in]
            n87 = case shown="12" "Camera Readout Mode" {
              tunnel: w361 -> [w372 w379]
              tunnel: [w371 w374] -> w354
              tunnel: w360 -> [w369 w384]
              tunnel: [w368 w384] -> w352
              frame 1, Default {
                n88 = local read "Exposure"() -> (w370:dbl)
                n89 = call <userlib>:"tm_setpropertyvalue.vi"("error in (no error)"=w369, "Value in"=w370, "Property ID"=u32 2031888, "Handle in"=w372) -> ("error out"=w368:errorcluster, "Handle out"=w371:u32)  [unwired: 6 in]
              }
              frame 12 {
                n90 = local read "Exposure"() -> (w383:dbl)
                n91 = local read "SVW"() -> (w381:i32)
                n92 = formula code="slitExpos=frameInter*LW/(LinesToReadout\n+10+LW);\nlineInter = slitExpos / LW;"("frameInter"=w383, "LW"="Slit Width / Lines", "LinesToReadout"=w381) -> ("slitExpos"=w375:dbl, "lineInter"=w378:dbl)
                n93 = call <userlib>:"tm_setpropertyvalue.vi"("Value in"=w378, "Property ID"=u32 4208720, "Handle in"=w379) -> ("Handle out"=w377:u32)  [unwired: 7 in, 1 out]
                n94 = call <userlib>:"tm_setpropertyvalue.vi"("Value in"=w375, "Property ID"=u32 2031888, "Handle in"=w377) -> ("Handle out"=w374:u32)  [unwired: 7 in, 1 out]
              }
            }
            n95 = call <userlib>:"tm_preparecapture.vi"("error in (no error)"=w352, "Capture mode"=w351, "Handle in"=w354) -> ("error out"=w347:errorcluster, "Buffer Info"=w353:T6, "Handle out"=w349:u32)  [unwired: 5 in, 1 out]
            n96 = call <userlib>:"tm_startcapture_b.vi"("error in (no error)"=w347, "Handle in"=w349) -> ("error out"=w346:errorcluster, "Handle out"=w348:u32)  [unwired: 8 in]
          }
          event "Ram Record": Value Change {
            n97 = event-data() -> ()  [unwired: 1 in, 5 out]
            n98 = case shown="True" "Ram Record" {
              tunnel: w398 -> [w402 w425]
              tunnel: w397 -> [w401 w422]
              tunnel: [w402 w408] -> w396
              tunnel: [w401 w410] -> w395
              tunnel: [w400 w409] -> w391
              tunnel: w390 -> [w400 _]
              tunnel: w388 -> [_ w413]
              tunnel: [_ w411] -> w387
              tunnel: w386 -> [_ w407]
              tunnel: w385 -> [_ w403]
              frame False {
              }
              frame True {
                w419 = 0 items=["Snap", "Sequence"] ("Capture mode")
                # "Max 2500"
                n99 = Flush Queue(queue=w413) -> (queue out=w412:refnum<queue>)  [unwired: 1 in, 2 out]
                n100 = call <userlib>:"tm_stopcapture.vi"("error in (no error)"=w425, "Handle in"=w422) -> ("error out"=w424:errorcluster, "Handle out"=w423:u32)  [unwired: 8 in]
                n101 = call <userlib>:"tm_unpreparecapture.vi"("error in (no error)"=w424, "Handle in"=w423) -> ("error out"=w420:errorcluster, "Handle out"=w421:u32)  [unwired: 8 in]
                n102 = call <userlib>:"tm_preparecapture.vi"("error in (no error)"=w420, "Frames"="Frames", "Capture mode"=w419, "Handle in"=w421) -> ("error out"=w418:errorcluster, "Buffer Info"=w416:T6, "Handle out"=w417:u32)  [unwired: 4 in, 1 out]
                n103 = Bundle By Name(cluster=w403, "State"=Stack_Track."Start Sequence", "Stack Number"=0, "Image"=w407) -> (w404:T3)
                n104 = Enqueue Element(queue=w412, element=w404) -> (queue out=w414:refnum<queue>)  [unwired: 2 in, 2 out]
                n105 = case shown="No Error" w418 {
                  selector: w418 -> [w450 w471]
                  tunnel: w417 -> [w449 w472]
                  tunnel: "Frames" -> [w445 _]
                  tunnel: [w430 w468] -> w410
                  tunnel: w416 -> [w446 _]
                  tunnel: [w429 w470] -> w408
                  tunnel: w414 -> [w444 w466]
                  tunnel: w403 -> [w443 _]
                  tunnel: [w428 w466] -> _
                  tunnel: [FALSE ("value") w480] -> w411
                  tunnel: [w427 w469] -> w409
                  frame No Error {
                    w435 = 1 items=["Snap", "Sequence"] ("Capture mode")
                    # "Frames in RAM"
                    n106 = call <userlib>:"tm_startcapture_b.vi"("error in (no error)"=w450, "Handle in"=w449) -> ("error out"=w447:errorcluster, "Handle out"=w448:u32)  [unwired: 8 in]
                    n107 = for {
                      N: w445 -> [_]
                      tunnel: w448 -> [w465]
                      tunnel: w447 -> [w464]
                      tunnel: w446 -> [w461]
                      tunnel: [w460] -> w441
                      tunnel: [w459] -> w440
                      tunnel: w444 -> [w457]
                      tunnel: Stack_Track."Collecting" ("Enum") -> [w455]
                      tunnel: w443 -> [w453]
                      tunnel: [w452] -> w434
                      i -> [w454]
                      n108 = call <userlib>:"tm_waitnextframe.vi"("error in (no error)"=w464, "Handle in"=w465) -> ("error out"=w462:errorcluster, "Frame Index"=→"Frame Index":i32, "Handle out"=w463:u32)  [unwired: 6 in, 1 out]
                      n109 = call <userlib>:"tm_getframe_a.vi"("error in (no error)"=w462, "Frame Index"=w454, "Buffer Info"=w461, "Handle in"=w463) -> ("error out"=w459:errorcluster, "Data 16"=w451:u16[][], "Handle out"=w460:u32)  [unwired: 3 in, 2 out]
                      n110 = Bundle By Name(cluster=w453, "State"=w455, "Stack Number"=w454, "Image"=w451) -> (w456:T3)
                      n111 = Enqueue Element(queue=w457, element=w456) -> (queue out=w452:refnum<queue>)  [unwired: 2 in, 2 out]
                    }
                    n112 = call <userlib>:"tm_stopcapture.vi"("error in (no error)"=w440, "Handle in"=w441) -> ("error out"=w438:errorcluster, "Handle out"=w439:u32)  [unwired: 8 in]
                    n113 = call <userlib>:"tm_unpreparecapture.vi"("error in (no error)"=w438, "Handle in"=w439) -> ("error out"=w437:errorcluster, "Handle out"=w436:u32)  [unwired: 8 in]
                    n114 = Enqueue Element(queue=w434, element=T3 {"State"=enum."End", "Stack Number"=0, "Image"=[]} ("input cluster")) -> (queue out=w428:refnum<queue>)  [unwired: 2 in, 2 out]
                    n115 = call <userlib>:"tm_preparecapture.vi"("error in (no error)"=w437, "Capture mode"=w435, "Handle in"=w436) -> ("error out"=w432:errorcluster, "Buffer Info"=w427:T6, "Handle out"=w431:u32)  [unwired: 5 in, 1 out]
                    n116 = call <userlib>:"tm_startcapture_b.vi"("error in (no error)"=w432, "Handle in"=w431) -> ("error out"=w429:errorcluster, "Handle out"=w430:u32)  [unwired: 8 in]
                  }
                  frame Error {
                    w475 = 1 items=["Snap", "Sequence"] ("Capture mode")
                    # "Prepare camera failure, likely too many frames in stack"
                    n117 = One Button Dialog(message="Too many frames in stack", button name ("OK")="OK") -> (true=w480:bool)
                    n118 = call <userlib>:"tm_stopcapture.vi"("error in (no error)"=w471, "Handle in"=w472) -> ("error out"=w478:errorcluster, "Handle out"=w479:u32)  [unwired: 8 in]
                    n119 = call <userlib>:"tm_unpreparecapture.vi"("error in (no error)"=w478, "Handle in"=w479) -> ("error out"=w477:errorcluster, "Handle out"=w476:u32)  [unwired: 8 in]
                    n120 = Enqueue Element(queue=w466, element=T3 {"State"=enum."Idle", "Stack Number"=0, "Image"=[]} ("input cluster")) -> ()  [unwired: 2 in, 3 out]
                    n121 = call <userlib>:"tm_preparecapture.vi"("error in (no error)"=w477, "Capture mode"=w475, "Handle in"=w476) -> ("error out"=w474:errorcluster, "Buffer Info"=w469:T6, "Handle out"=w473:u32)  [unwired: 5 in, 1 out]
                    n122 = call <userlib>:"tm_startcapture_b.vi"("error in (no error)"=w474, "Handle in"=w473) -> ("error out"=w470:errorcluster, "Handle out"=w468:u32)  [unwired: 8 in]
                  }
                }
              }
            }
          }
          event "HardDisk Record": Value Change {
            n123 = event-data() -> ()  [unwired: 1 in, 5 out]
            n124 = case shown="True" "HardDisk Record" {
              tunnel: w495 -> [w498 w514]
              tunnel: w494 -> [w497 w511]
              tunnel: [w498 w501] -> w493
              tunnel: [w497 w503] -> w492
              tunnel: [w496 w502] -> w488
              tunnel: w487 -> [w496 _]
              tunnel: w485 -> [_ w499]
              tunnel: [_ w504] -> w484
              frame False {
              }
              frame True {
                w508 = 0 items=["Snap", "Sequence"] ("Capture mode")
                # "Max 50"
                n125 = call <userlib>:"tm_stopcapture.vi"("error in (no error)"=w514, "Handle in"=w511) -> ("error out"=w513:errorcluster, "Handle out"=w512:u32)  [unwired: 8 in]
                n126 = call <userlib>:"tm_unpreparecapture.vi"("error in (no error)"=w513, "Handle in"=w512) -> ("error out"=w509:errorcluster, "Handle out"=w510:u32)  [unwired: 8 in]
                n127 = call <userlib>:"tm_preparecapture.vi"("error in (no error)"=w509, "Frames"="Frames", "Capture mode"=w508, "Handle in"=w510) -> ("error out"=w507:errorcluster, "Buffer Info"=w505:T6, "Handle out"=w506:u32)  [unwired: 4 in, 1 out]
                n128 = case shown="No Error" w507 {
                  selector: w507 -> [w539 w552]
                  tunnel: w506 -> [w525 w553]
                  tunnel: [w528 w549] -> w503
                  tunnel: w505 -> [w536 _]
                  tunnel: [w527 w551] -> w501
                  tunnel: [FALSE ("value") w561] -> w504
                  tunnel: [w526 w550] -> w502
                  tunnel: "Frames" -> [w522 _]
                  tunnel: w499 -> [w516 w547]
                  frame No Error {
                    w531 = 1 items=["Snap", "Sequence"] ("Capture mode")
                    n129 = call <userlib>:"tm_startrecorder.vi"("frames"=w522, "File"="Temp", "Handle in"=w525) -> ("Handle out"=w524:u32)  [unwired: 7 in, 1 out]
                    n130 = call <userlib>:"tm_startcapture_b.vi"("error in (no error)"=w539, "Handle in"=w524) -> ("error out"=w537:errorcluster, "Handle out"=w538:u32)  [unwired: 8 in]
                    n131 = while {
                      tunnel: w538 -> [w545]
                      tunnel: w537 -> [w544]
                      tunnel: w536 -> [_]
                      tunnel: [w546] -> w534
                      tunnel: w522 -> [w541]
                      stop <- w542 stop-if-true
                      n132 = Wait (ms)(milliseconds to wait=u32 50) -> ()  [unwired: 1 out]
                      n133 = call <userlib>:"tm_getrecorderstatus.vi"("error in (no error)"=w544, "Handle"=w545) -> ("error out"=w546:errorcluster, "Count"=w540:i32)  [unwired: 6 in, 2 out]
                      n134 = Equal?(x=w540, y=w541) -> (x = y?=w542:bool)
                    }
                    n135 = call <userlib>:"tm_stopcapture.vi"("error in (no error)"=w534) -> ("error out"=w521:errorcluster, "Handle out"=w520:u32)  [unwired: 9 in]
                    n136 = call <userlib>:"tm_stoprecorder.vi"("error in (no error)"=w521, "Handle in"=w520) -> ("error out"=w518:errorcluster, "Handle out"=w519:u32)  [unwired: 8 in]
                    n137 = Enqueue Element(queue=w516, element=T3 {"State"=enum."Read Disk", "Stack Number"=0, "Image"=[]}, error in (no error)=w518) -> (error out=w517:errorcluster)  [unwired: 1 in, 2 out]
                    n138 = call <userlib>:"tm_unpreparecapture.vi"("error in (no error)"=w517, "Handle in"=w519) -> ("error out"=w533:errorcluster, "Handle out"=w532:u32)  [unwired: 8 in]
                    n139 = call <userlib>:"tm_preparecapture.vi"("error in (no error)"=w533, "Capture mode"=w531, "Handle in"=w532) -> ("error out"=w530:errorcluster, "Buffer Info"=w526:T6, "Handle out"=w529:u32)  [unwired: 5 in, 1 out]
                    n140 = call <userlib>:"tm_startcapture_b.vi"("error in (no error)"=w530, "Handle in"=w529) -> ("error out"=w527:errorcluster, "Handle out"=w528:u32)  [unwired: 8 in]
                  }
                  frame Error {
                    w556 = 1 items=["Snap", "Sequence"] ("Capture mode")
                    # "Prepare camera failure, likely too many frames in stack"
                    n141 = One Button Dialog(message="Too many frames in stack", button name ("OK")="OK") -> (true=w561:bool)
                    n142 = call <userlib>:"tm_stopcapture.vi"("error in (no error)"=w552, "Handle in"=w553) -> ("error out"=w559:errorcluster, "Handle out"=w560:u32)  [unwired: 8 in]
                    n143 = call <userlib>:"tm_unpreparecapture.vi"("error in (no error)"=w559, "Handle in"=w560) -> ("error out"=w558:errorcluster, "Handle out"=w557:u32)  [unwired: 8 in]
                    n144 = Enqueue Element(queue=w547, element=T3 {"State"=enum."STOP", "Stack Number"=0, "Image"=[]} ("input cluster")) -> ()  [unwired: 2 in, 3 out]
                    n145 = call <userlib>:"tm_preparecapture.vi"("error in (no error)"=w558, "Capture mode"=w556, "Handle in"=w557) -> ("error out"=w555:errorcluster, "Buffer Info"=w550:T6, "Handle out"=w554:u32)  [unwired: 5 in, 1 out]
                    n146 = call <userlib>:"tm_startcapture_b.vi"("error in (no error)"=w555, "Handle in"=w554) -> ("error out"=w551:errorcluster, "Handle out"=w549:u32)  [unwired: 8 in]
                  }
                }
              }
            }
          }
          event "Scan Mode": Value Change {
            w564 = u32 4211872 items=["SENSOR MODE"=4212128, "CCD MODE"=4212384, "READOUT MODE"=4211872, "ACTIVE VIEW INDEX"=4343136, "BITS PER CHANNEL"=4342976, "IMAGE PIXEL TYPE"=4343296, "BINNING"=4215968, "EXPOSURE TIME"=2049184, "CONTRAST GAIN"=3163312, "CONTRAST OFFSET"=3163328, "LIGHT MODE"=2114720, "SENSITIVITY"=2114992, "PHOTON IMAGING MODE"=2115200, "HIGH DYNAMIC RANGE MODE"=3163360, "WHITE BALANCE"=3163568, "TEMPERATURE"=2115232, "TEMPERATURE TARGET"=2115264, "SENSOR COOLER FAN"=2115296, "LINEBUNDLE HEIGHT"=4212192, "MECHANICAL SHUTTER"=2115488, "BACK FOCUS POSITION"=8422304, "TRIGGER CONNECTOR"=1066432, "TRIGGER SOURCE"=1066144, "OUTPUT TRIGGER SOURCE"=1852576, "TRIGGER GLOBAL EXPOSURE"=2049680, "FIRST TRIGGER BEHAVIOR"=2049696, "CHANNEL SYNC"=1852352, "READOUT DIRECTION"=4211904, "PRE HSYNC COUNT"=1852704] ("Parameter")
            w579 = 1 items=["Snap", "Sequence"] ("Capture mode")
            n147 = event-data() -> ("NewVal"=w569:dbl)  [unwired: 1 in, 2 out]
            n148 = call <userlib>:"tm_stopcapture.vi"("error in (no error)"=w580, "Handle in"=w581) -> ("error out"=w582:errorcluster, "Handle out"=w583:u32)  [unwired: 8 in]
            n149 = call <userlib>:"tm_unpreparecapture.vi"("error in (no error)"=w582, "Handle in"=w583) -> ("error out"=w567:errorcluster, "Handle out"=w568:u32)  [unwired: 8 in]
            n150 = call <userlib>:"tm_setparameter_a.vi"("error in (no error)"=w567, "Value in"=w569, "Parameter"=w564, "Handle in"=w568) -> ("error out"=w566:errorcluster, "Handle out"=w565:u32)  [unwired: 6 in]
            n151 = call <userlib>:"tm_getparameter_a.vi"("error in (no error)"=w566, "Parameter"=w564, "Handle in"=w565) -> ("error out"=w572:errorcluster, "Value out"=w571:dbl, "Handle out"=w570:u32)  [unwired: 6 in]
            n152 = local write "SMD"(w571) -> ()
            n153 = call <userlib>:"tm_preparecapture.vi"("error in (no error)"=w572, "Capture mode"=w579, "Handle in"=w570) -> ("error out"=w577:errorcluster, "Buffer Info"=w574:T6, "Handle out"=w578:u32)  [unwired: 5 in, 1 out]
            n154 = call <userlib>:"tm_startcapture_b.vi"("error in (no error)"=w577, "Handle in"=w578) -> ("error out"=w576:errorcluster, "Handle out"=w575:u32)  [unwired: 8 in]
          }
          event "Binning": Value Change {
            w588 = u32 4215968 items=["BINNING"=4215968, "BITS PER CHANNEL"=2, "ACTIVE VIEW INDEX"=3, "CCD MODE"=4, "SENSOR MODE"=5, "READOUT MODE"=6, "EXPOSURE TIME"=7, "CONTRAST GAIN"=8, "CONTRAST OFFSET"=9, "LIGHT MODE"=10, "SENSITIVITY"=11, "WHITE BALANCE"=12, "PHOTON IMAGING MODE"=13, "HIGH DYNAMIC RANGE MODE"=14, "TRIGGER SOURCE"=15, "TRIGGER ACTIVE"=16, "TRIGGER MODE"=17, "TRIGGER POLARITY"=18, "TRIGGER GLOBAL EXPOSURE"=19, "FIRST TRIGGER BEHAVIOR"=20, "TRIGGER TIMES"=21, "OUTPUT TRIGGER POLARITY"=22, "OUTPUT TRIGGER DELAY"=23, "OUTPUT TRIGGER PERIOD"=24, "TEMPERATURE"=25, "TEMPERATURE TARGET"=26, "SENSOR COOLER FAN"=27, "MECHANICAL SHUTTER"=28, "BACK FOCUS POSITION"=29, "FRAMEBUNDLE MODE"=30, "FRAMEBUNDLE NUMBER"=31, "LINEBUNDLE HEIGHT"=32, "TRIGGER CONNECTOR"=33, "IMAGE PIXEL TYPE"=34, "OUTPUT TRIGGER KIND"=35, "READOUT DIRECTION"=36, "CHANNEL SYNC"=37] ("Parameter")
            w627 = 1 items=["Snap", "Sequence"] ("Capture mode")
            n155 = event-data() -> ("NewVal"=w589:u16)  [unwired: 1 in, 2 out]
            n156 = call <userlib>:"tm_stopcapture.vi"("error in (no error)"=w596, "Handle in"=w597) -> ("error out"=w594:errorcluster, "Handle out"=w595:u32)  [unwired: 8 in]
            n157 = call <userlib>:"tm_unpreparecapture.vi"("error in (no error)"=w594, "Handle in"=w595) -> ("error out"=w590:errorcluster, "Handle out"=w587:u32)  [unwired: 8 in]
            n158 = call <userlib>:"tm_setparameter_a.vi"("error in (no error)"=w590, "Value in"=w589, "Parameter"=w588, "Handle in"=w587) -> ("error out"=w591:errorcluster, "Handle out"=w592:u32)  [unwired: 6 in]
            n159 = call <userlib>:"tm_getarea_a.vi"("error in (no error)"=w591, "Handle in"=w592) -> ("error out"=w615:errorcluster, "V Offset"=w617:T5, "H Offset"=w616:T5, "Handle out"=w614:u32, "H Width"=w618:T5, "V Width"=w619:T5)  [unwired: 4 in]
            n160 = Unbundle By Name(w616) -> ("Value"=w610:i32, "Minimum"=w613:i32, "Maximum"=w612:i32, "Increment"=w611:i32)
            n161 = Unbundle By Name(w617) -> ("Value"=w600:i32, "Minimum"=w609:i32, "Maximum"=w608:i32, "Increment"=w607:i32)
            n162 = Unbundle By Name(w618) -> ("Value"=w599:i32, "Minimum"=w606:i32, "Maximum"=w605:i32, "Increment"=w604:i32)
            n163 = Unbundle By Name(w619) -> ("Value"=w598:i32, "Minimum"=w603:i32, "Maximum"=w602:i32, "Increment"=w601:i32)
            n164 = property on="H Offset" class="DigNum (strict)"("Value"=w610, "Minimum"=w613, "Maximum"=w612, "Increment"=w611) -> ()  [unwired: 2 in, 2 out]
            n165 = property on="V Offset" class="DigNum (strict)"("Value"=w600, "Minimum"=w609, "Maximum"=w608, "Increment"=w607) -> ()  [unwired: 2 in, 2 out]
            n166 = property on="H Width" class="DigNum (strict)"("Value"=w599, "Minimum"=w606, "Maximum"=w605, "Increment"=w604) -> ()  [unwired: 2 in, 2 out]
            n167 = property on="V Width" class="DigNum (strict)"("Value"=w598, "Minimum"=w603, "Maximum"=w602, "Increment"=w601) -> ()  [unwired: 2 in, 2 out]
            n168 = local write "SHO"(w610) -> ()
            n169 = local write "SVO"(w600) -> ()
            n170 = local write "SHW"(w599) -> ()
            n171 = local write "SVW"(w598) -> ()
            n172 = call <userlib>:"tm_preparecapture.vi"("error in (no error)"=w615, "Capture mode"=w627, "Handle in"=w614) -> ("error out"=w625:errorcluster, "Buffer Info"=w622:T6, "Handle out"=w626:u32)  [unwired: 5 in, 1 out]
            n173 = call <userlib>:"tm_startcapture_b.vi"("error in (no error)"=w625, "Handle in"=w626) -> ("error out"=w624:errorcluster, "Handle out"=w623:u32)  [unwired: 8 in]
          }
          event "H Offset", "H Width", "V Offset", "V Width": Value Change {
            w672 = 1 items=["Snap", "Sequence"] ("Capture mode")
            n174 = event-data() -> ()  [unwired: 1 in, 4 out]
            n175 = call <userlib>:"tm_stopcapture.vi"("error in (no error)"=w634, "Handle in"=w635) -> ("error out"=w632:errorcluster, "Handle out"=w633:u32)  [unwired: 8 in]
            n176 = local read "H Offset"() -> (w638:i32)
            n177 = local read "H Width"() -> (w639:i32)
            n178 = local read "V Offset"() -> (w640:i32)
            n179 = local read "V Width"() -> (w637:i32)
            n180 = call <userlib>:"tm_unpreparecapture.vi"("error in (no error)"=w632, "Handle in"=w633) -> ("error out"=w630:errorcluster, "Handle out"=w631:u32)  [unwired: 8 in]
            n181 = Bundle("H Offset"=w638, "V Offset"=w640, "H Width"=w639, "V Width"=w637) -> (w636:T7)  [unwired: 1 in]
            n182 = call <userlib>:"tm_setarea.vi"("error in (no error)"=w630, "Sub Region"=w636, "Handle in"=w631) -> ("error out"=w641:errorcluster, "Handle out"=w642:u32)  [unwired: 7 in]
            n183 = call <userlib>:"tm_getarea_a.vi"("error in (no error)"=w641, "Handle in"=w642) -> ("error out"=w660:errorcluster, "V Offset"=w662:T5, "H Offset"=w661:T5, "Handle out"=w659:u32, "H Width"=w663:T5, "V Width"=w664:T5)  [unwired: 4 in]
            n184 = Unbundle By Name(w661) -> ("Value"=w655:i32, "Minimum"=w658:i32, "Maximum"=w657:i32, "Increment"=w656:i32)
            n185 = Unbundle By Name(w662) -> ("Value"=w645:i32, "Minimum"=w654:i32, "Maximum"=w653:i32, "Increment"=w652:i32)
            n186 = Unbundle By Name(w663) -> ("Value"=w644:i32, "Minimum"=w651:i32, "Maximum"=w650:i32, "Increment"=w649:i32)
            n187 = Unbundle By Name(w664) -> ("Value"=w643:i32, "Minimum"=w648:i32, "Maximum"=w647:i32, "Increment"=w646:i32)
            n188 = property on="H Offset" class="DigNum (strict)"("Value"=w655, "Minimum"=w658, "Maximum"=w657, "Increment"=w656) -> ()  [unwired: 2 in, 2 out]
            n189 = property on="V Offset" class="DigNum (strict)"("Value"=w645, "Minimum"=w654, "Maximum"=w653, "Increment"=w652) -> ()  [unwired: 2 in, 2 out]
            n190 = property on="H Width" class="DigNum (strict)"("Value"=w644, "Minimum"=w651, "Maximum"=w650, "Increment"=w649) -> ()  [unwired: 2 in, 2 out]
            n191 = property on="V Width" class="DigNum (strict)"("Value"=w643, "Minimum"=w648, "Maximum"=w647, "Increment"=w646) -> ()  [unwired: 2 in, 2 out]
            n192 = local write "SHO"(w655) -> ()
            n193 = local write "SVO"(w645) -> ()
            n194 = local write "SHW"(w644) -> ()
            n195 = local write "SVW"(w643) -> ()
            n196 = call <userlib>:"tm_preparecapture.vi"("error in (no error)"=w660, "Capture mode"=w672, "Handle in"=w659) -> ("error out"=w670:errorcluster, "Buffer Info"=w667:T6, "Handle out"=w671:u32)  [unwired: 5 in, 1 out]
            n197 = call <userlib>:"tm_startcapture_b.vi"("error in (no error)"=w670, "Handle in"=w671) -> ("error out"=w669:errorcluster, "Handle out"=w668:u32)  [unwired: 8 in]
          }
        }
        n198 = Unbundle By Name(w184) -> ("status"=w197:bool)
        n199 = Compound Arithmetic op=OR(w197, "stop", w178) -> (w196:bool)
      }
      n200 = while {
        tunnel: w8 -> [w104]
        shift-right: [w100] -> _
        shift-left: _ -> [w98]
        shift-right: [w96] -> _
        shift-left: _ -> [w97]
        shift-right: [w94] -> _
        shift-left: _ -> [w90]
        stop <- w99 stop-if-true
        n201 = Dequeue Element(queue=w104) -> (element=w103:T3, timed out?=w91:bool)  [unwired: 2 in, 2 out]
        n202 = Unbundle By Name(w103) -> ("State"=w102:T1, "Stack Number"=w101:i32, "Image"=w92:u16[][])
        "State" <- w102
        n203 = case shown="True" w91 {
          tunnel: w92 -> [w106 w108]
          tunnel: [w106 w107] -> w93
          tunnel: [w105 w108] -> w94
          tunnel: w90 -> [w105 w107]
          frame False {
          }
          frame True {
          }
        }
        "Image" <- w93
        n204 = case shown="\"Start Sequence\"" w102 {
          tunnel: w101 -> [_ _ _ _ _ _]
          tunnel: [w111 w128 _ _ _ _] -> w100
          tunnel: w98 -> [_ w129 w135 _ _ _]
          tunnel: [FALSE _ _ _ TRUE _] -> w99
          tunnel: w93 -> [w109 w130 _ _ _ _]
          tunnel: w97 -> [_ w127 w133 w145 w170 w172]
          tunnel: [w112 w126 w134 w141 w170 w172] -> w96
          tunnel: "Path" -> [w115 _ _ w147 _ _]
          frame "Start Sequence" {
            # "Public tiff library"
            # "Get path and open file"
            n205 = Equal?(x=w115, y=path "") -> (x = y?=w117:bool)
            n206 = case shown="True" w117 {
              tunnel: w115 -> [w119 _]
              tunnel: [w119 w122] -> w114
              frame False {
              }
              frame True {
                n207 = call "File Dialog"("pattern (all files)"=".tiff", "pattern label"="Tiff Image") -> ("selected path"=w122:path)  [unwired: 10 in, 3 out]
              }
            }
            n208 = case shown="False" "AutoIncrement" {
              tunnel: w114 -> [w123 w125]
              tunnel: [w123 w124] -> w110
              frame False {
              }
              frame True {
                n209 = call "4Digit File Incrementer.vi"("path"=w125) -> ("appended path"=w124:path)  [unwired: 10 in]
              }
            }
            n210 = call-poly "CTIFFNewFileAndStyle.vi"("image"=w109, "output_file"=w110) -> ("error"=w112:errorcluster, "CTIFF"=w111:i64)  [unwired: 8 in]
            n211 = local write "Path"(w110) -> ()
          }
          frame "Collecting" {
            # "Add Image to write scan line"
            n212 = call-poly "CTIFFAddNewPage.vi"("error"=w127, "image"=w130, "CTIFF"=w129) -> ("error"=w126:errorcluster, "CTIFF"=w128:i64)  [unwired: 7 in]
            n213 = property on="Ram Record" class="Bool (strict)"("DisabledEnum"=T2."Disabled and Grayed Out" ("Disabled"), "BoolText.Text"="Saving" ("Boolean Text.Text")) -> ()  [unwired: 2 in, 2 out]
          }
          frame "End" {
            (unwired) FALSE
            # "Close image file, reset capturing button"
            n214 = call "CTIFFWriteAndClose.vi"("error"=w133, "CTIFF"=w135) -> ("error"=w134:errorcluster)  [unwired: 9 in]
            n215 = property on="Ram Record" class="Bool (strict)"("BoolText.Text"="OK" ("Boolean Text.Text"), "DisabledEnum"=T2."Enabled" ("Disabled")) -> ()  [unwired: 2 in, 2 out]
          }
          frame "Read Disk" {
            n216 = local read "Temp"() -> (w142:path)
            n217 = call <userlib>:"tm_opendcimgfile.vi"("Path"=w142) -> ("Total Frames"=w148:i32, "File Handle"=w149:u32)  [unwired: 8 in, 1 out]
            n218 = for {
              N: w148 -> [_]
              tunnel: w147 -> [w157]
              shift-right: [w155] -> w143
              shift-left: i64 0 ("CTIFF") -> [w156]
              tunnel: [w154] -> w144
              tunnel: w145 -> [w153]
              shift-right: [w159] -> w138
              shift-left: w149 -> [w160]
              i -> [w151]
              n219 = Equal To 0?(x=w151) -> (x = 0?=w158:bool)
              n220 = call <userlib>:"tm_getdcimgframe.vi"("error in (no error)"=w153, "Frame Index"=w151, "File Handle in"=w160) -> ("error out"=w152:errorcluster, "Data"=w150:u16[][], "File Handle out"=w159:u32)  [unwired: 5 in, 1 out]
              n221 = local write "Image"(w150) -> ()
              n222 = case shown="True" w158 {
                tunnel: w157 -> [_ w169]
                tunnel: w150 -> [w161 w168]
                tunnel: w156 -> [w165 _]
                tunnel: [w164 w167] -> w155
                tunnel: [w163 w166] -> w154
                tunnel: w152 -> [w162 _]
                frame False {
                  n223 = call-poly "CTIFFAddNewPage.vi"("error"=w162, "image"=w161, "CTIFF"=w165) -> ("error"=w163:errorcluster, "CTIFF"=w164:i64)  [unwired: 7 in]
                }
                frame True {
                  n224 = call-poly "CTIFFNewFileAndStyle.vi"("image"=w168, "output_file"=w169) -> ("error"=w166:errorcluster, "CTIFF"=w167:i64)  [unwired: 8 in]
                }
              }
              "Frame Index" <- w151
            }
            n225 = call "CTIFFWriteAndClose.vi"("error"=w144, "CTIFF"=w143) -> ("error"=w140:errorcluster)  [unwired: 9 in]
            n226 = call <userlib>:"tm_closedcimgfile.vi"("error in (no error)"=w140, "File Handle"=w138) -> ("error out"=w139:errorcluster)  [unwired: 9 in]
            n227 = Delete(path (use dialog)=w142, error in=w139) -> (error out=w141:errorcluster)  [unwired: 3 in, 2 out]
          }
          frame "STOP" {
          }
          frame "Idle" {
          }
        }
      }
      n228 = call <userlib>:"tm_stopcapture.vi"("error in (no error)"=w57, "Handle in"=w58) -> ("error out"=w54:errorcluster, "Handle out"=w55:u32)  [unwired: 8 in]
      n229 = call <userlib>:"tm_unpreparecapture.vi"("error in (no error)"=w54, "Handle in"=w55) -> ("error out"=w53:errorcluster, "Handle out"=w56:u32)  [unwired: 8 in]
      n230 = call <userlib>:"tm_closecamera.vi"("error in (no error)"=w53, "Handle in"=w56) -> ("error out"=w87:errorcluster)  [unwired: 9 in]
      n231 = call <userlib>:"tm_deinitialize.vi"("error in (no error)"=w87) -> ("error out"=w86:errorcluster)  [unwired: 10 in]
    }
  }
  "error out" <- w3
